vi "Write to Pivots.vi"   [LabVIEW 2014]
uses:
  Begin/Global RefNums.vi
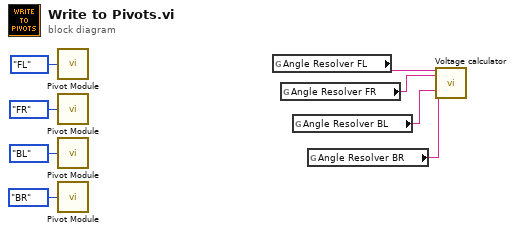
[diagram p0: block diagram]
diagram:
  n1 = call "Pivot Module.vi"("pivot"=enum16{"FL", "FR", "BL", "BR"}."FL") -> ()
  n2 = call "Pivot Module.vi"("pivot"=enum16{"FL", "FR", "BL", "BR"}."FR") -> ()
  n3 = call "Pivot Module.vi"("pivot"=enum16{"FL", "FR", "BL", "BR"}."BL") -> ()
  n4 = call "Pivot Module.vi"("pivot"=enum16{"FL", "FR", "BL", "BR"}."BR") -> ()
  n5 = global read "Global RefNums.vi" "Angle Resolver FL"() -> (w4:string)
  n6 = global read "Global RefNums.vi" "Angle Resolver FR"() -> (w3:string)
  n7 = global read "Global RefNums.vi" "Angle Resolver BL"() -> (w2:string)
  n8 = global read "Global RefNums.vi" "Angle Resolver BR"() -> (w1:string)
  n9 = call "Voltage calculator.vi"("ROT FL"=w4, "ROT FR"=w3, "ROT BL"=w2, "ROT BR"=w1) -> ()  [unwired: 8 in, 8 out]
